vi "niScope Get Frequency Response.vi"(0 "instrument handle":refnum<k15>, 5 "channels":string="0", 11 "error in":errorcluster) -> (4 "instrument handle out":refnum<k15>, 6 "frequencies":dbl[](array[numeric]), 8 "magnitudes":dbl[](array[numeric]), 10 "phases":dbl[](array[numeric]), 14 "numberOfFrequencies":i32, 15 "error out":errorcluster)   [LabVIEW 2011]
doc: "Gets the frequency response of the digitizer for the current configurations of the channel attributes. This VI can be used only with high-speed digitizers that support onboard signal processing (OSP)."
uses:
  niScope_32.dll
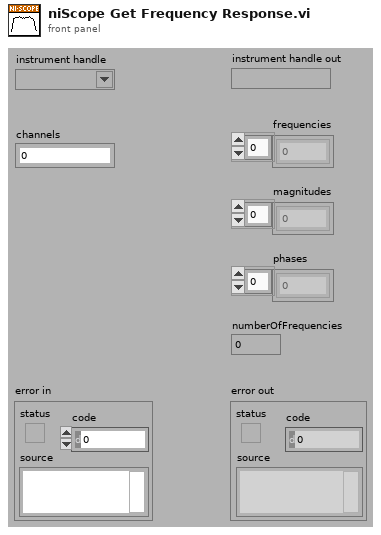
[diagram p1: front panel]
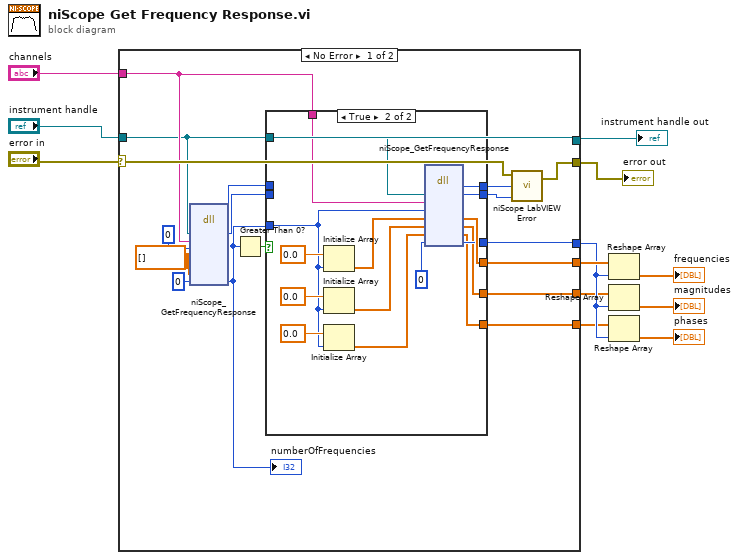
[diagram p0: block diagram]
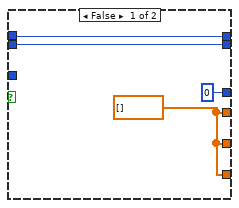
[diagram p2: hidden frame]
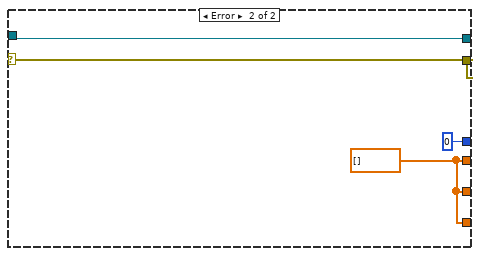
[diagram p3: hidden frame]
diagram:
  n1 = case shown="No Error" "error in" {
    selector: "error in" -> [w26 w51]
    tunnel: [w29 w51] -> w12
    tunnel: "instrument handle" -> [w13 w53]
    tunnel: [w13 w53] -> w11
    tunnel: [w20 w50] -> w7
    tunnel: [w17 0 ("actualSamples")] -> w6
    tunnel: "channels" -> [w24 _]
    tunnel: [w19 w50] -> w5
    tunnel: [w18 w50] -> w4
    frame No Error {
      w25 = dbl[] [] ("frequencies")
      n2 = dll-call lib="niScope_*.*" fn="niScope_GetFrequencyResponse"("instrument handle"=w13, "channel"=w24, "bufferSize"=0, "frequencies"=w25, "amplitudes"=w25, "phases"=w25, "numberOfFrequencies"=0) -> ("status"=w14:i32, "instrument handle"=w16:u32, "numberOfFrequencies"=w15:i32)  [unwired: 8 in, 2 out]
      "numberOfFrequencies" <- w15
      n3 = Greater Than 0?(x=w15) -> (x > 0?=w21:bool)
      n4 = case shown="True" w21 {
        tunnel: [w30 w49] -> w28
        tunnel: [w31 w48] -> w27
        tunnel: w24 -> [_ w44]
        tunnel: w13 -> [_ w43]
        tunnel: w15 -> [_ w39]
        tunnel: [w33 w37] -> w20
        tunnel: [0 ("numberOfFrequencies") w36] -> w17
        tunnel: [w33 w35] -> w19
        tunnel: [w33 w34] -> w18
        tunnel: w16 -> [w31 _]
        tunnel: w14 -> [w30 _]
        frame False {
          w33 = dbl[] [] ("frequencies")
        }
        frame True {
          n5 = Initialize Array(0.0 ("Element Data"), w39) -> (w42:dbl[])
          n6 = Initialize Array(0.0 ("Element Data"), w39) -> (w41:dbl[])
          n7 = Initialize Array(0.0 ("Element Data"), w39) -> (w40:dbl[])
          n8 = dll-call lib="niScope_*.*" fn="niScope_GetFrequencyResponse"("instrument handle"=w43, "channel"=w44, "bufferSize"=w39, "frequencies"=w42, "amplitudes"=w41, "phases"=w40, "numberOfFrequencies"=0) -> ("status"=w49:i32, "instrument handle"=w48:u32, "frequencies"=w37:dbl[], "amplitudes"=w35:dbl[], "phases"=w34:dbl[], "numberOfFrequencies"=w36:i32)  [unwired: 5 in, 2 out]
        }
      }
      n9 = call <instrlib>:"niScope LabVIEW Error.vi"("instrument handle"=w27, "niScope error code (0)"=w28, "error in (no error)"=w26) -> ("error out"=w29:errorcluster)  [unwired: 2 in]
    }
    frame Error {
      w50 = dbl[] [] ("frequencies")
    }
  }
  "error out" <- w12
  "instrument handle out" <- w11
  n10 = Reshape Array(w7, w6) -> (→"frequencies":dbl[])
  n11 = Reshape Array(w5, w6) -> (→"magnitudes":dbl[])
  n12 = Reshape Array(w4, w6) -> (→"phases":dbl[])
